vi "主画面.vi"() -> ()   [LabVIEW 2016]
uses:
  <vilib>/Utility/config.llb/Read Key (String).vi
  <vilib>/Utility/config.llb/NI_LVConfig.lvlib
  data/FreeMem.dll
panel:
  in  "全屏":T1
  out "站点名称":string="站点名称"
  out "时间显示":string="2017-05-09 10:50:42"
  out "Version":string="Version:1.0.0"
  in  "主画面菜单":enum32{"首页", "数据查询", "运维调试", "系统设置"}(xcontrol)
  # "一 体 化 微 型 水 质 监 测 站"
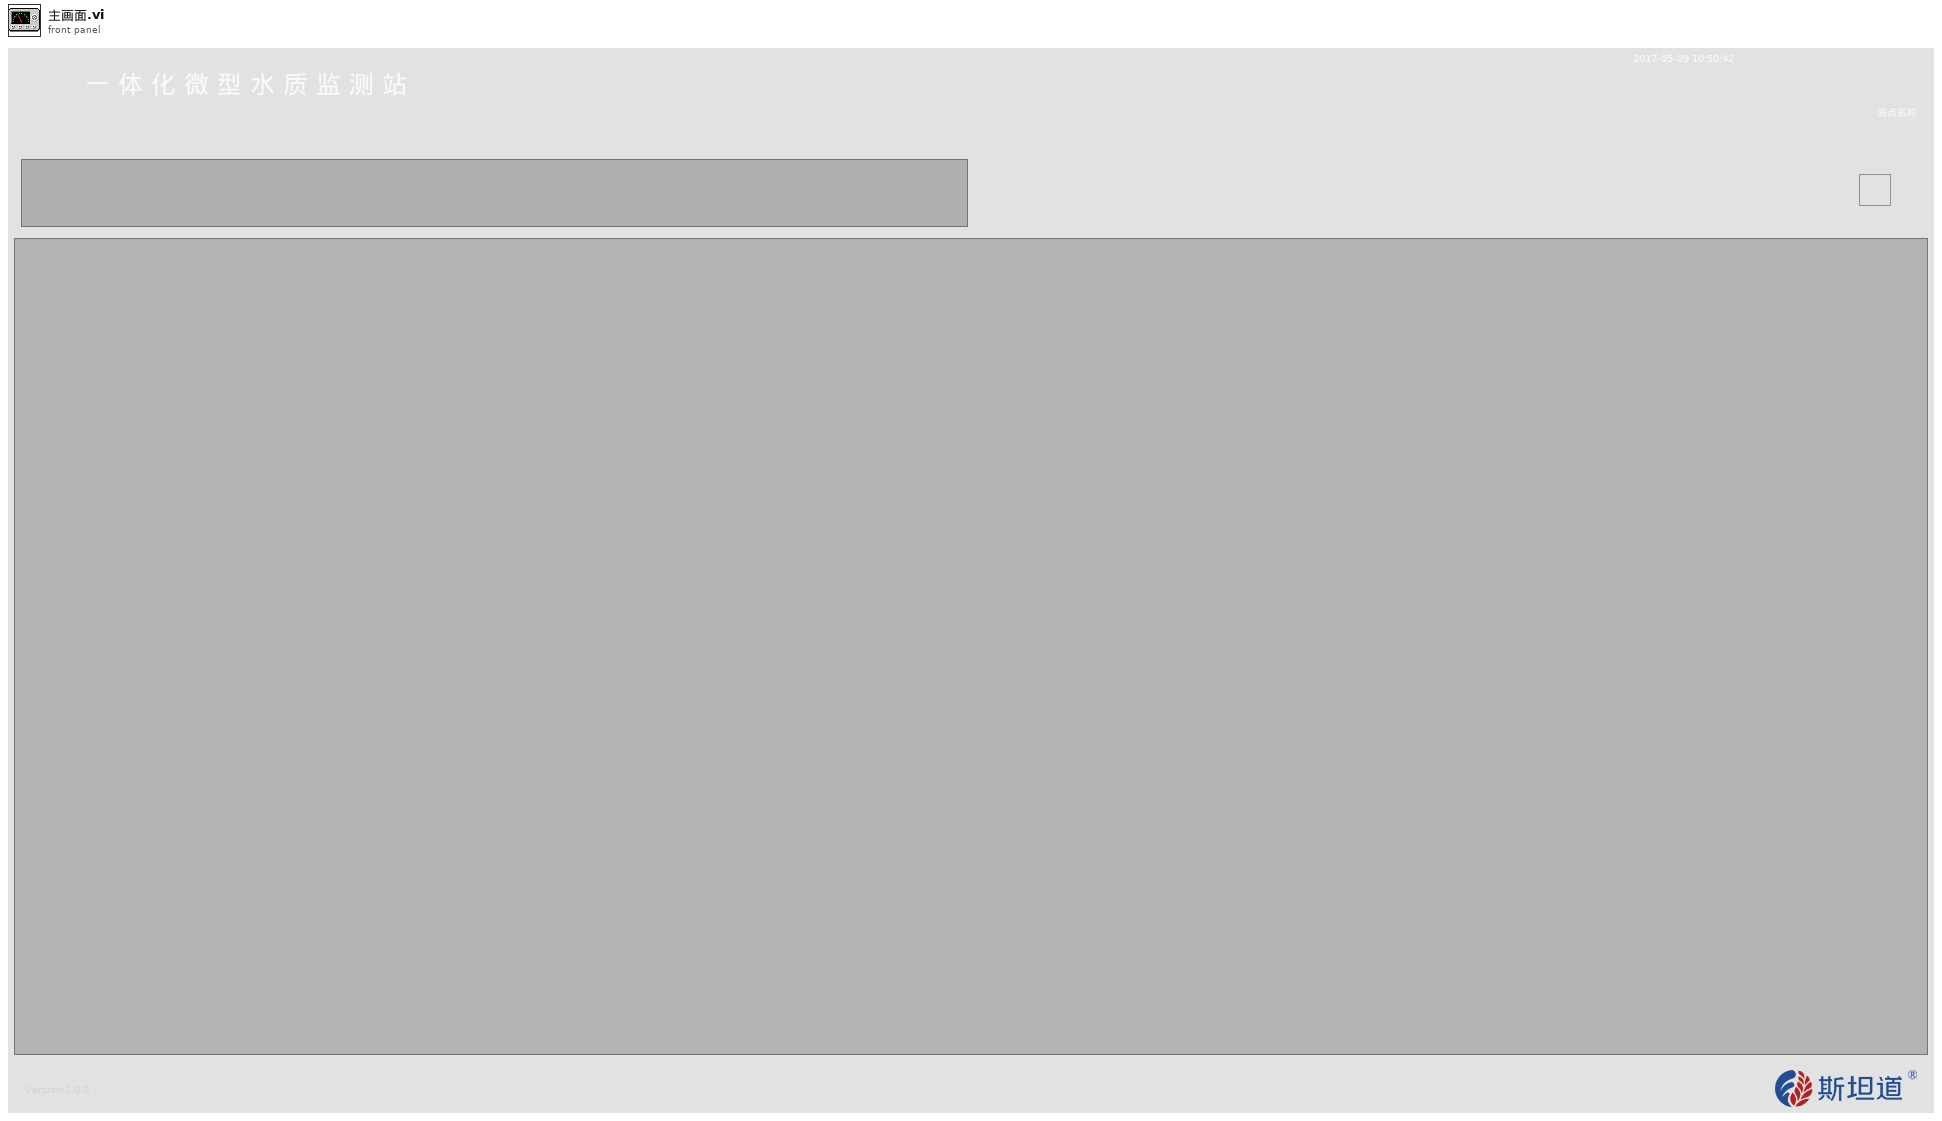
[diagram p1: front panel]
types:
  T1 = typedef "全屏按钮.ctl" = bool
  T2 = cluster{"时间标识":timestamp, "设备":string, "日志信息":string, "流程参数":string}
  T3 = enum32{"invalid app kind", "Development System", "Run Time System", "Student Edition", "Embedded LabVIEW", "Evaluation", "Custom"}
  T4 = typedef "NI_LVConfig.lvlib/Config Data RefNum.ctl" = refnum<k1>
  T5 = enum32{"Bad", "Idle", "Run top level", "Running"}
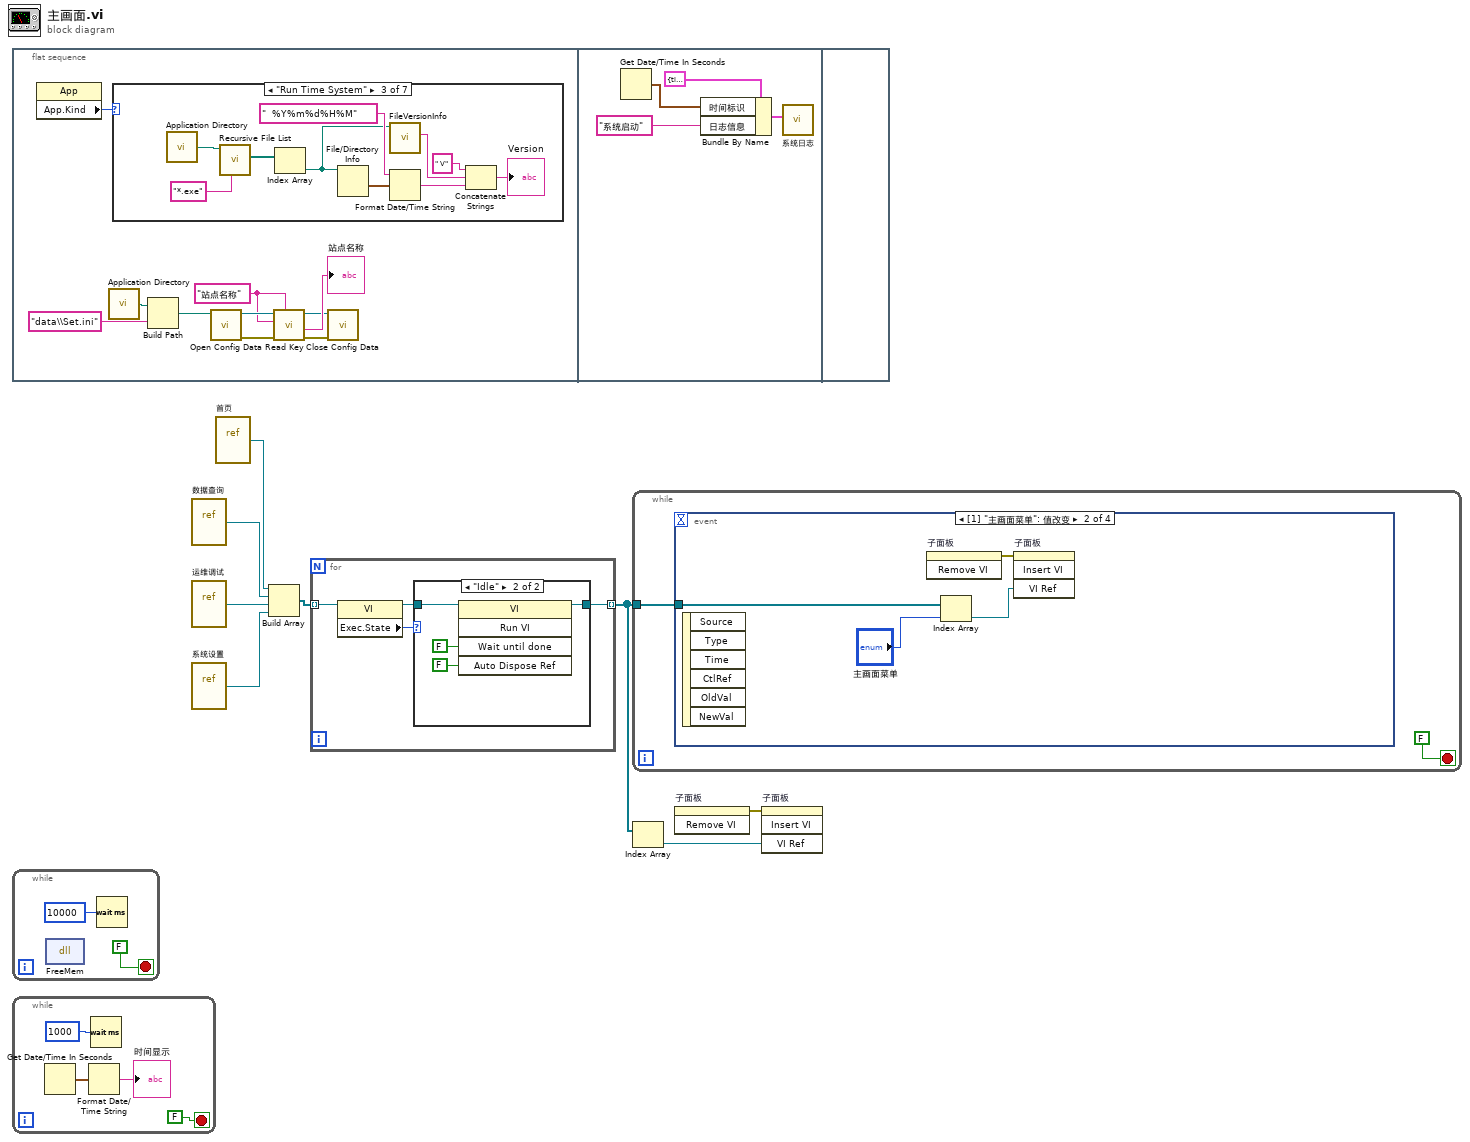
[diagram p0: block diagram]
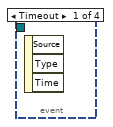
[diagram p9: hidden frame]
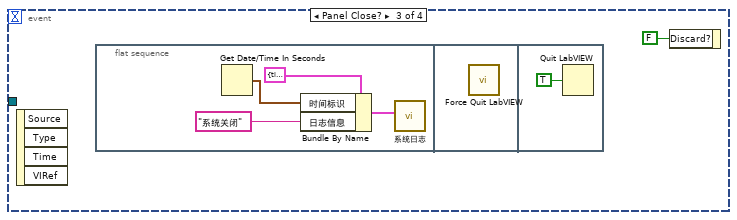
[diagram p10: hidden frame]
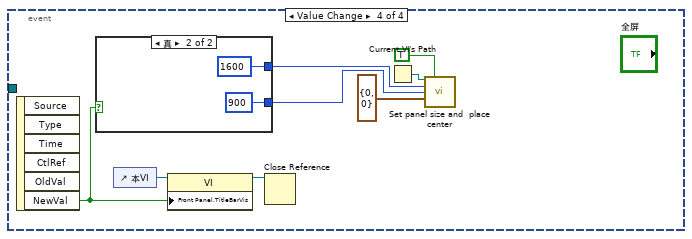
[diagram p11: hidden frame]
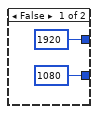
[diagram p12: hidden frame]
diagram:
  n1 = flat-sequence {
    frame #0 {
      w9 = "站点名称" ("section")
      n2 = property class="App"() -> ("App.Kind"=w18:T3)  [unwired: 2 in, 2 out]
      n3 = call <vilib>:"Application Directory.vi"() -> ("Application Directory"=w12:path)
      n4 = case shown="\"Run Time System\"" w18 {
        frame "invalid app kind" {
        }
        frame "Development System", Default {
        }
        frame "Run Time System" {
          n5 = call <vilib>:"Application Directory.vi"() -> ("Application Directory"=w20:path)
          n6 = call <vilib>:"Recursive File List.vi"("pattern"="*.exe", "Folder Path"=w20) -> ("All Files in Dir"=w21:path[])  [unwired: 5 in, 4 out]
          n7 = Index Array(array=w21) -> (element=w19:path)  [unwired: 1 in]
          n8 = File/Directory Info(path=w19) -> (last mod=w25:timestamp)  [unwired: 1 in, 6 out]
          n9 = call <vilib>:"FileVersionInfo.vi"("Application Path in"=w19) -> ("File Version Info"=w27:string)  [unwired: 7 in, 3 out]
          n10 = Format Date/Time String(time format string (%c)="  %Y%m%d%H%M" ("时间格式字符串(%c)"), seconds (now)=w25) -> (date/time string=w23:string)  [unwired: 1 in]
          n11 = Concatenate Strings(" V" ("字符串"), w27, w23) -> (→"Version":string)
        }
        frame "Student Edition" {
        }
        frame "Embedded LabVIEW" {
        }
        frame "Evaluation" {
        }
        frame "Custom" {
        }
      }
      n12 = Build Path(base path=w12, name or relative path="data\\Set.ini" ("名称或相对路径")) -> (appended path=w10:path)
      n13 = call <vilib>:"Open Config Data.vi"("configuration file path"=w10) -> ("error out"=w14:errorcluster, "refnum"=w17:T4)  [unwired: 8 in, 1 out]
      n14 = call-poly <vilib>:"Read Key.vi"("section"=w9, "error in (no error)"=w14, "key"=w9, "refnum"=w17) -> ("error out"=w13:errorcluster, "value"=→"站点名称":string, "refnum out"=w15:T4)  [unwired: 4 in, 1 out]
      n15 = call <vilib>:"Close Config Data.vi"("error in (no error)"=w13, "refnum"=w15) -> ()  [unwired: 8 in, 2 out]
    }
    frame #1 {
      n16 = Get Date/Time In Seconds() -> (seconds since 1Jan1904=w30:timestamp)
      n17 = Bundle By Name(cluster=T2 {"时间标识"=timestamp(0 s since 1904-01-01), "设备"="系统", "日志信息"="", "流程参数"=""} ("data in"), "时间标识"=w30, "日志信息"="系统启动") -> (w31:T2)
      n18 = call "系统日志.vi"("data in"=w31) -> ()  [unwired: 11 in]
    }
    frame #2 {
    }
  }
  n19 = while {
    stop <- FALSE stop-if-true
    n20 = dll-call lib="PTH2qabs CUsers\nAdministrator\tDocuments集成项目一体站项目样版一体站项目dataFreeMem.dll" fn="FreeMem"() -> ()  [unwired: 4 in, 2 out]
    n21 = Wait (ms)(milliseconds to wait=u32 10000 ("等待时间（毫秒）")) -> ()  [unwired: 1 out]
  }
  n22 = while {
    stop <- FALSE stop-if-true
    n23 = Get Date/Time In Seconds() -> (seconds since 1Jan1904=w35:timestamp)
    n24 = Format Date/Time String(seconds (now)=w35) -> (date/time string=→"时间显示":string)  [unwired: 2 in]
    n25 = Wait (ms)(milliseconds to wait=u32 1000 ("等待时间（毫秒）")) -> ()  [unwired: 1 out]
  }
  n26 = vi-ref "数据查询.vi"() -> (w4:refnum<vi>)
  n27 = vi-ref "运维调试.vi"() -> (w3:refnum<vi>)
  n28 = vi-ref "系统设置.vi"() -> (w2:refnum<vi>)
  n29 = vi-ref "首页.vi"() -> (w5:refnum<vi>)
  n30 = Build Array(w5, w4, w3, w2) -> (w1:refnum<vi>[])
  n31 = for {
    tunnel: w1 -> [w42] mode=indexing
    tunnel: [w39] -> w7 mode=indexing
    n32 = property class="VI"(reference=w42) -> (reference out=w40:refnum<vi>, "Exec.State"=w41:T5)  [unwired: 1 in, 1 out]
    n33 = case shown="\"Idle\"" w41 {
      tunnel: w40 -> [w43 w45]
      tunnel: [w43 w44] -> w39
      frame "Bad", Default {
      }
      frame "Idle" {
        n34 = invoke class="VI" method="Run VI"(reference=w45, "Wait until done"=FALSE ("结束前等待"), "Auto Dispose Ref"=FALSE ("自动销毁引用")) -> (reference out=w44:refnum<vi>)  [unwired: 2 in, 4 out]
      }
    }
  }
  n35 = while {
    tunnel: w7 -> [w48]
    stop <- FALSE stop-if-true
    n36 = event shown="[1] \"主画面菜单\": 值改变" {
      selector: _ -> [_ _ _ _]
      dyn-events: _ -> [_ _ _ _]
      timeout: _ -> [_ _ _ _]
      tunnel: w48 -> [_ w52 _ _]
      event Timeout {
        n37 = event-data() -> ()  [unwired: 1 in, 3 out]
      }
      event "主画面菜单": Value Change {
        n38 = event-data() -> ()  [unwired: 1 in, 6 out]
        n39 = invoke on="子面板" class="SubPnl" method="Remove VI"() -> (error out=w50:errorcluster)  [unwired: 3 in, 2 out]
        n40 = Index Array(array=w52, index="主画面菜单") -> (element=w51:refnum<vi>)
        n41 = invoke on="子面板" class="SubPnl" method="Insert VI"(error in=w50, "VI Ref"=w51) -> ()  [unwired: 2 in, 4 out]
      }
      event Panel Close? {
        n42 = event-data() -> ()  [unwired: 1 in, 4 out]
        n43 = flat-sequence {
          frame #0 {
            n44 = Get Date/Time In Seconds() -> (seconds since 1Jan1904=w57:timestamp)
            n45 = Bundle By Name(cluster=T2 {"时间标识"=timestamp(0 s since 1904-01-01), "设备"="系统", "日志信息"="", "流程参数"=""} ("data in"), "时间标识"=w57, "日志信息"="系统关闭") -> (w56:T2)
            n46 = call "系统日志.vi"("data in"=w56) -> ()  [unwired: 11 in]
          }
          frame #1 {
            n47 = call "Force Quit LabVIEW.vi"() -> ()  [unwired: 10 in, 2 out]
          }
          frame #2 {
            n48 = Quit LabVIEW(quit? (T)=TRUE ("退出？(T)")) -> ()
          }
        }
        n49 = event-data("Discard?"=FALSE ("放弃？")) -> ()  [unwired: 1 in, 1 out]
      }
      event Value Change {
        n50 = event-data() -> ("NewVal"=w62:T1)  [unwired: 1 in, 5 out]
        n51 = case shown="真" w62 {
          tunnel: [1920 ("Panel Width") 1600 ("Panel Width")] -> w61
          tunnel: [1080 ("Panel Height") 900 ("Panel Height")] -> w60
          frame False {
          }
          frame True {
          }
        }
        n52 = control-ref of="本VI"() -> (w67:refnum<vi>)
        n53 = property class="VI"(reference=w67, "Front Panel.TitleBarVis"=w62) -> (reference out=w63:refnum<vi>)  [unwired: 1 in, 1 out]
        n54 = Close Reference(reference=w63) -> ()  [unwired: 1 in, 1 out]
        n55 = Current VI's Path() -> (path=w66:path)
        n56 = call "Set panel size and  place center.vi"("Path"=w66, "Close Reference (false)"=TRUE, "Panel Width"=w61, "Panel Height"=w60, "FP.Origin in(H & V)"=cluster{"Horizontal":i16, "Vertical":i16} {"Horizontal"=0, "Vertical"=0}) -> ()  [unwired: 6 in, 5 out]
      }
    }
  }
  n57 = Index Array(array=w7) -> (element=w6:refnum<vi>)  [unwired: 1 in]
  n58 = invoke on="子面板" class="SubPnl" method="Remove VI"() -> (error out=w8:errorcluster)  [unwired: 3 in, 2 out]
  n59 = invoke on="子面板" class="SubPnl" method="Insert VI"(error in=w8, "VI Ref"=w6) -> ()  [unwired: 2 in, 4 out]
